vi "4155C Config SamplingI Measurements v2.0.vi"(0 "VISA session":refnum<visa-resource-name>, 1 "Num Points":i16=1 min=1 max=1001, 2 "Sample I - Probe 3 (Disabled)":u32(ring)=2 items=["SMU1  ", "SMU2  ", "SMU3  ", "SMU4  ", "SMU5  ", "SMU6  "], 3 "Display on/off":bool, 5 "Sample I - Source/Common":u32(ring) items=["SMU1  ", "SMU2  ", "SMU3  ", "SMU4  ", "SMU5  ", "SMU6  "], 7 "Sample I - Drain/Gate":u32(ring)=1 items=["SMU1  ", "SMU2  ", "SMU3  ", "SMU4  ", "SMU5  ", "SMU6  "], 9 "Sampling interval":dbl min=0.0 max=100000000000.0 format="%.6f", 10 "Standby":T1, 11 "error in (no error)":errorcluster, 12 "Timings":T2={"integration time"=0, "Short/Long integration time"=0.00064, "hold time (sec)"=0.0, "delay time (sec)"=0.0, "Step Time (0 disables)"=0.0, "sweep method"=0, "Pulse period"=0.005, "Base voltage"=0.0, "Pulse width"=0.0005} {"Pulse width" min=0.0005 max=0.1 step=0.0001 format="%.4f"; "Base voltage" min=-100.0 max=100.0 format="%^.4e"; "Pulse period" min=0.005 max=1.0 step=0.0001 format="%.4f"; "sweep method" items=["Continuous", "Pulsed"]; "Step Time (0 disables)" format="%.2f"; "delay time (sec)" min=0.0 format="%.4f"; "hold time (sec)" min=0.0 format="%.4f"; "Short/Long integration time" min=0.0 format="%^.0e"; "integration time" scale=0.0..2.0}, 13 "Sample I - Probe 4 (Disabled)":u32(ring)=3 items=["SMU1  ", "SMU2  ", "SMU3  ", "SMU4  ", "SMU5  ", "SMU6  "], 14 "Sample time":dbl min=0.0 max=100000000000.0 format="%.2f") -> (4 "dup VISA resource name":refnum<visa-resource-name>, 15 "error out":errorcluster)   [LabVIEW 2016]
doc: "This VI configures the primary sweep source (VAR1) for a sweep mode measurement. \n* This VI does not perform error checking on MEASUREMENT MODE or UNIT TYPE of VAR1, therefore it is the application programmer's responsibility to make certain this VI is used in the proper mode."
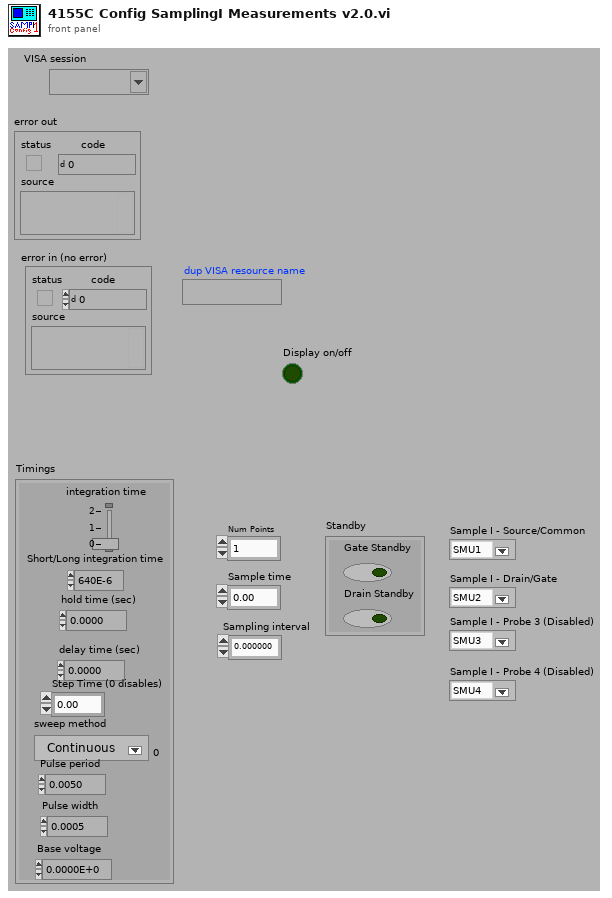
[diagram p1: front panel]
types:
  T1 = cluster{"Gate Standby":bool, "Drain Standby":bool}
  T2 = cluster{"integration time":u32, "Short/Long integration time":dbl, "hold time (sec)":dbl, "delay time (sec)":dbl, "Step Time (0 disables)":dbl, "sweep method":u16, "Pulse period":dbl, "Base voltage":dbl, "Pulse width":dbl}
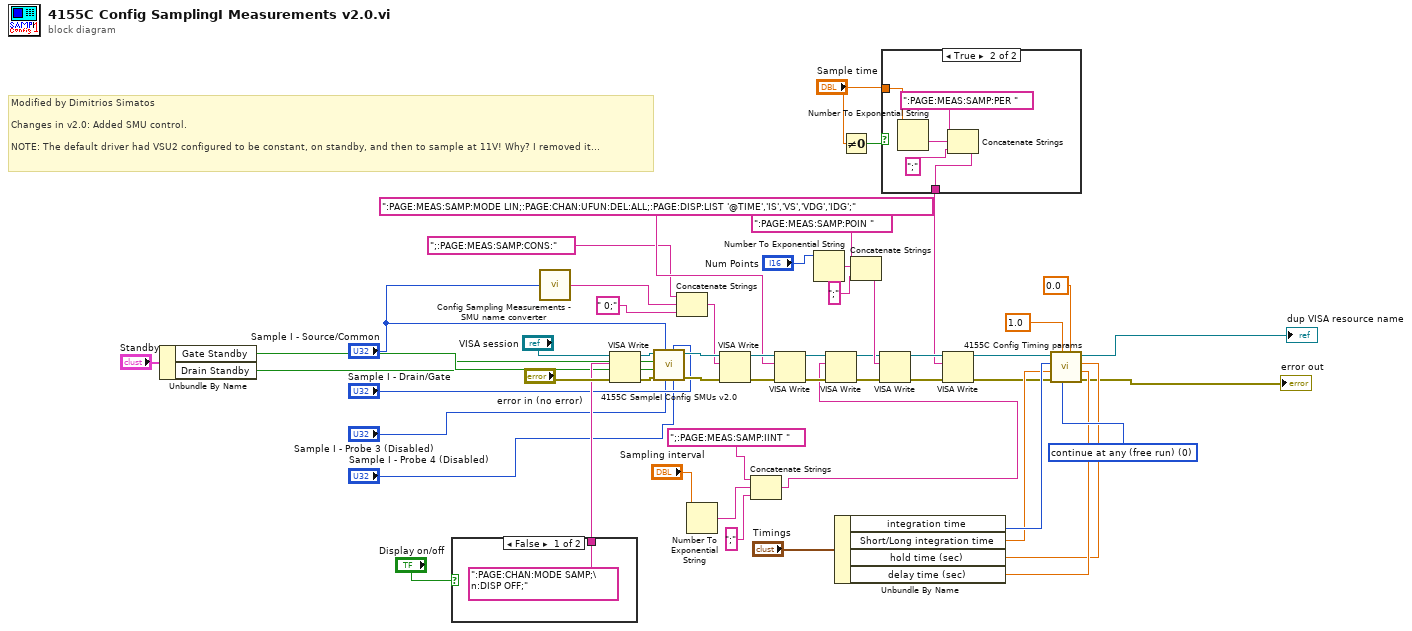
[diagram p0: block diagram]
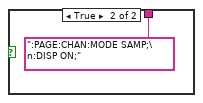
[diagram p2: hidden frame]
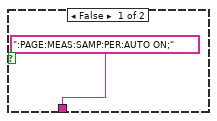
[diagram p3: hidden frame]
diagram:
  w51 = u8 0 items=["continue at any (free run)", "stop at any abnorm", "stop at compliance"] ("stop condition (free run:0)")
  # "Modified by Dimitrios Simatos\n\nChanges in v2.0: Added SMU control.\n\nNOTE: The default driver had VSU2 configured to be constant, on standby, and then to sample at 11V! Why? I removed it..."
  n1 = Unbundle By Name("Standby") -> ("Gate Standby"=w2:bool, "Drain Standby"=w1:bool)
  n2 = case shown="False" "Display on/off" {
    tunnel: [":PAGE:CHAN:MODE SAMP;\n:DISP OFF;" ("write buffer (\"\")") ":PAGE:CHAN:MODE SAMP;\n:DISP ON;" ("write buffer (\"\")")] -> w22
    frame False {
    }
    frame True {
    }
  }
  n3 = call "Config Sampling Measurements - SMU name converter.vi"("unit to configure"="Sample I - Source/Common") -> ("SMU to be configured"=w9:string)
  n4 = VISA Write(VISA resource name="VISA session", write buffer=w22, error in (no error)="error in (no error)") -> (VISA resource name out=w40:refnum<visa-resource-name>, error out=w39:errorcluster)  [unwired: 1 out]
  n5 = call "4155C SampleI Config SMUs v2.0.vi"("Sample I - Probe 4 (Disabled)"="Sample I - Probe 4 (Disabled)", "Sample I - Drain/Gate"="Sample I - Drain/Gate", "Sample I - Probe 3 (Disabled)"="Sample I - Probe 3 (Disabled)", "Sample I - Source/Common"="Sample I - Source/Common", "error in (no error)"=w39, "Gate Standby"=w2, "Drain Standby"=w1, "VISA resource name in"=w40) -> ("error out"=w38:errorcluster, "VISA Resource Name out"=w37:refnum<visa-resource-name>)  [unwired: 2 in]
  n6 = Concatenate Strings(";:PAGE:MEAS:SAMP:CONS:" ("write buffer (\"\")"), w9, " 0;" ("write buffer (\"\")")) -> (w11:string)
  n7 = Number To Exponential String(number="Sampling interval") -> (E-format string=w21:string)  [unwired: 3 in]
  n8 = VISA Write(VISA resource name=w37, write buffer=w11, error in (no error)=w38) -> (VISA resource name out=w53:refnum<visa-resource-name>, error out=w52:errorcluster)  [unwired: 1 out]
  n9 = Concatenate Strings(";:PAGE:MEAS:SAMP:IINT ", w21, ";" ("Substring")) -> (w14:string)
  n10 = VISA Write(VISA resource name=w53, write buffer=":PAGE:MEAS:SAMP:MODE LIN;:PAGE:CHAN:UFUN:DEL:ALL;:PAGE:DISP:LIST '@TIME','IS','VS','VDG','IDG';", error in (no error)=w52) -> (VISA resource name out=w13:refnum<visa-resource-name>, error out=w17:errorcluster)  [unwired: 1 out]
  n11 = Number To Exponential String(number="Num Points") -> (E-format string=w35:string)  [unwired: 3 in]
  n12 = VISA Write(VISA resource name=w13, write buffer=w14, error in (no error)=w17) -> (VISA resource name out=w15:refnum<visa-resource-name>, error out=w16:errorcluster)  [unwired: 1 out]
  n13 = Unbundle By Name("Timings") -> ("integration time"=w48:u32, "Short/Long integration time"=w43:dbl, "hold time (sec)"=w49:dbl, "delay time (sec)"=w50:dbl)
  n14 = Not Equal To 0?(x="Sample time") -> (x != 0?=w29:bool)
  n15 = Concatenate Strings(":PAGE:MEAS:SAMP:POIN " ("write buffer (\"\")"), w35, ";" ("Substring")) -> (w31:string)
  n16 = VISA Write(VISA resource name=w15, write buffer=w31, error in (no error)=w16) -> (VISA resource name out=w28:refnum<visa-resource-name>, error out=w27:errorcluster)  [unwired: 1 out]
  n17 = case shown="True" w29 {
    tunnel: "Sample time" -> [_ w60]
    tunnel: [":PAGE:MEAS:SAMP:PER:AUTO ON;" w57] -> w24
    frame False {
    }
    frame True {
      n18 = Number To Exponential String(number=w60) -> (E-format string=w61:string)  [unwired: 3 in]
      n19 = Concatenate Strings(":PAGE:MEAS:SAMP:PER " ("Substring"), w61, ";" ("Substring")) -> (w57:string)
    }
  }
  n20 = VISA Write(VISA resource name=w28, write buffer=w24, error in (no error)=w27) -> (VISA resource name out=w25:refnum<visa-resource-name>, error out=w26:errorcluster)  [unwired: 1 out]
  n21 = call "4155C Config Timing params.vi"("delay time (sec)"=w50, "hold time (sec)"=w49, "Step Time (0 disables)"=0.0, "stop condition (free run:0)"=w51, "wait time parameter"=1.0, "error in (no error)"=w26, "Short/Long integration time"=w43, "integration time"=w48, "VISA session"=w25) -> ("error out"=→"error out":errorcluster, "dup VISA resource name"=→"dup VISA resource name":refnum<visa-resource-name>)  [unwired: 1 in]
